vi "Get Full Error Details Text.vi"(1 "Error Message":string, 2 "Error Code":i32) -> (0 "Full Error Details Text":string)   [LabVIEW 2016, in "Error Manager.lvlib"]
doc: "This VI generates a \"Full Error Details\" string, which can be displayed to the user and/or logged to the error log file."
uses:
  Error Manager.lvlib
panel:
  # "Development\nControls or indicators that are useful for development or testing, but which are not outputs of the VI."
  # "Input\nInputs to the VI"
  # "Output\nOutputs of the VI"
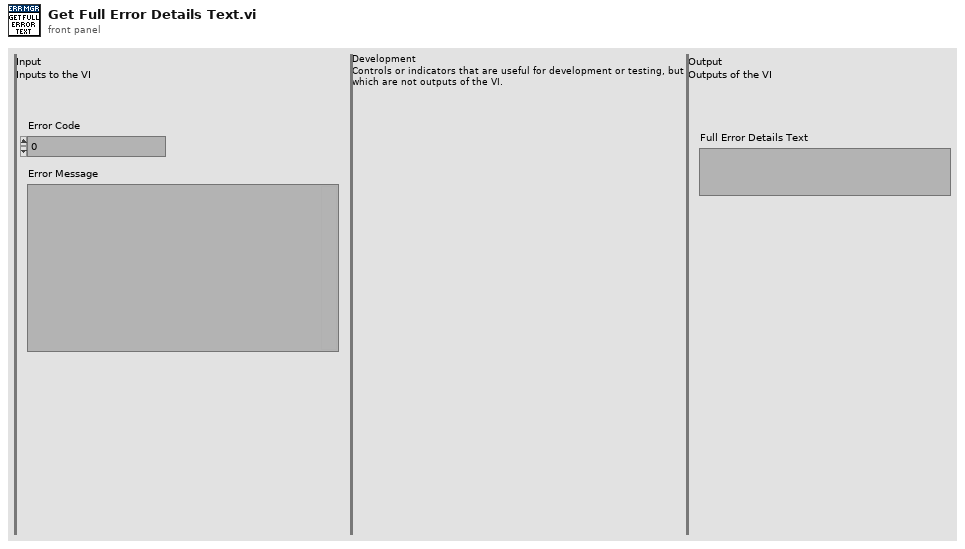
[diagram p1: front panel]
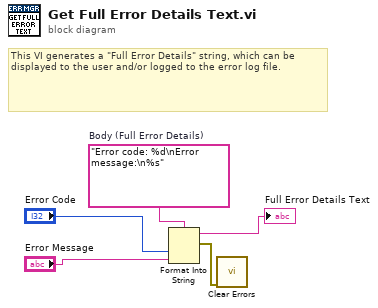
[diagram p0: block diagram]
diagram:
  w5 = "Error code: %d\nError message:\n%s"  # Body (Full Error Details)
  # "This VI generates a \"Full Error Details\" string, which can be displayed to the user and/or logged to the error log file."
  n1 = Format Into String(format string=w5, "Error Code", "Error Message") -> (resulting string=→"Full Error Details Text":string, error out=w4:errorcluster)  [unwired: 2 in]
  n2 = call <vilib>:"Clear Errors.vi"("error in (no error)"=w4) -> ()  [unwired: 5 in, 2 out]
